vi "AxisUI.vi"(10 "CardNumber":i32, 11 "IO Card Type":T1) -> ()   [LabVIEW 2019]
uses:
  IO Folder/IO_VI/IOCtrl/Ctrl/IO Card_Type.ctl
  Ctrl/right2.ctl
  Ctrl/left2.ctl
  Ctrl/Up2.ctl
  Ctrl/down2.ctl
  Ctrl/Clock2.ctl
  Ctrl/CClock2.ctl
  Ctrl/Teach2.ctl
  Ctrl/Move.ctl
  Ctrl/EmgStop.ctl
  Ctrl/SearchHome.ctl
  <vilib>/Utility/miscctls.llb/LVPointTypeDef.ctl
  LLB/Message/Ctrl/MsgDataInput.ctl
  LLB/Message/Ctrl/MsgPageSelect.ctl
  LLB/Message/Ctrl/LogType.ctl
  IO Folder/IO_VI/IOCtrl/Ctrl/DMC1000B_1 SelectOutput.ctl
  Axis_Class/AxisCard.lvclass
  Axis_Class/DMC 1000B/DMC_1000B.lvclass
  C:/Users/VIC/Desktop/204J1/204J1/System/Function/Axis/Axis_Class/AxisCard.lvclass
  Axis_Class/SubVI/Axis Motion/Axis_Jump Point.vi
  Axis_Class/SubVI/Axis Motion/Axis_Go Point.vi
  Axis_Class/SubVI/Axis Motion/Axis_Go Related.vi
  Axis_Class/SubVI/Axis Motion/Axis_Go Home.vi
  LLB/Commonly VI.lvlib
  LLB/Message/MsgShowAndLog.lvlib
  LLB/DMC1000B/Dmc1000/Dmc1000.lvlib
panel:
  out "Axis Q":refnum<queue>
  out "Axis Q Name":string
  in  "Tab Control":enum32{"Page 1", "Page 2"}(tab)
  in  "Save Button":bool
  out "Actioning":bool
  in  "Btn_EmgStop":T2
  in  "Tab Control 2":enum32{"Control", "PointEdit", "Parameter"}(tab)
  out "Home Finish":T3 caption="Home"
  in  "SearchHome":T4
  in  "JogDistance":cluster{"X":dbl, "Y":dbl, "Z":dbl, "U":dbl}={"X"=10.0, "Y"=10.0, "Z"=10.0, "U"=10.0} caption="寸動距離/JogDistance" {"U" min=0.01 max=100.0 format="%#.3f"; "Z" min=0.01 max=100.0 format="%#.3f"; "Y" min=0.01 max=100.0 format="%#.3f"; "X" min=0.01 max=100.0 format="%#.3f"}
  in  "Btn_Move":T5
  in  "PointSelect":u16(ring) caption="點位選擇/PointSelect" items=["P0 - HM", "P1 - Mark1"]
  in  "Btn_Teach":T6
  in  "Move Action":enum16{"Jump", "Go"}(ring) caption="移動方式/Mode"
  in  "Current Position":cluster{"X":dbl, "Y":dbl, "Z":dbl, "U":dbl} caption="當前位置/Current Position" {"U" format="%#.3f"; "Z" format="%#.3f"; "Y" format="%#.3f"; "X" format="%#.3f"}
  in  "Jog Distance Select":enum32{"Long", "Middle", "Short"}(radio)=enum."Middle" caption="寸動間距選擇(mm)/Jog Distance Select(mm)"
  in  "Jog":T13 caption="寸動/Jog"
  in  "AxisSpeed Basic":T14(array[cluster])=[{"AxisName"="Axis_0", "Accel"=0.5, "Deaccel"=0.5, "Speed"=40000.0, "Sramp"=0.4}, {"AxisName"="Axis_1", "Accel"=0.5, "Deaccel"=0.5, "Speed"=40000.0, "Sramp"=0.4}, {"AxisName"="Axis_2", "Accel"=0.5, "Deaccel"=0.5, "Speed"=40000.0, "Sramp"=0.4}, {"AxisName"="Axis_3", "Accel"=0.5, "Deaccel"=0.5, "Speed"=40000.0, "Sramp"=0.4}]
  in  "RobotPoint":string[][](table)
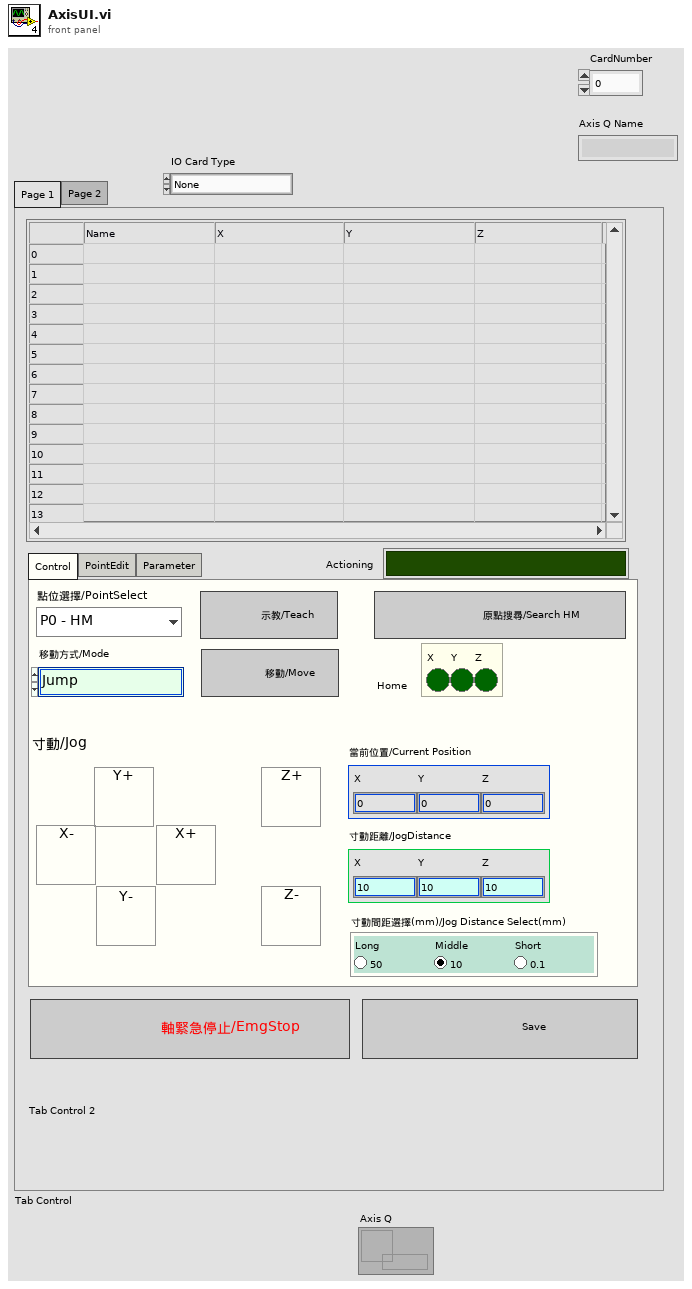
[diagram p1: front panel]
types:
  T1 = typedef "IO Card_Type.ctl" = enum16{"None", "Unidaq32", "6480", "2410C-64", "Zan", "DMC1000B", "16InOut", "Robot", "DMC3600"}
  T2 = typedef "EmgStop.ctl" = bool
  T3 = cluster{"Axis_0":bool, "Axis_1":bool, "Axis_2":bool, "Axis_3":bool}
  T4 = typedef "SearchHome.ctl" = bool
  T5 = typedef "Move.ctl" = bool
  T6 = typedef "Teach2.ctl" = bool
  T7 = typedef "right2.ctl" = bool
  T8 = typedef "left2.ctl" = bool
  T9 = typedef "Up2.ctl" = bool
  T10 = typedef "down2.ctl" = bool
  T11 = typedef "Clock2.ctl" = bool
  T12 = typedef "CClock2.ctl" = bool
  T13 = cluster{"X+":T7, "X-":T8, "Y+":T9, "Y-":T10, "Z+":T9, "Z-":T10, "U+":T11, "U-":T12}
  T14 = cluster{"AxisName":string, "Accel":dbl, "Deaccel":dbl, "Speed":dbl, "Sramp":dbl}[]
  T15 = typedef "LVPointTypeDef.ctl" = cluster{"Horizontal":i16, "Vertical":i16}
  T16 = typedef "MsgDataInput.ctl" = cluster{"MsgPageSelect":T17, "LogType":T18, "Msg":string, "Time":string}
  T17 = typedef "MsgShowAndLog.lvlib/MsgPageSelect.ctl" = enum16{"System", "Comm", "IO", "Action", "Alarm"}
  T18 = typedef "MsgShowAndLog.lvlib/LogType.ctl" = enum16{"Auto", "Manual", "Handshake", "Error"}
  T19 = enum16{"Initial", "Load", "Save", "Read", "WriteSpeed", "WritePoint"}
  T20 = cluster{"Move Action":enum16{"Jump", "Go"}, "RingText.Text":string}
  T21 = cluster{"Move Action":enum16{"Jump", "Go"}, "trimmed string":string}
  T22 = cluster{"[0]":dbl, "[1]":dbl, "[2]":dbl, "[3]":dbl}
  T23 = cluster{"Home Finish[0]":bool, "Home Finish[1]":bool, "Home Finish[2]":bool, "Home Finish[3]":bool}
  T24 = cluster{"Current Position[0]":dbl, "Current Position[1]":dbl, "Current Position[2]":dbl, "Current Position[3]":dbl}
  T25 = typedef "DMC1000B_1 SelectOutput.ctl" = enum16{"M_Out0預備", "M_OUT01蜂鳴器", "M_OUT02紅燈", "M_OUT03綠燈", "M_OUT04黃燈", "M_OUT05上頂固定位氣缸電磁閥", "M_OUT06到料阻擋氣缸電磁閥", "M_OUT07向前機台發出要料#1信號", "M_OUT08向前機台發出要料#2信號", "M_OUT09向後機台發出有料#3信號", "M_OUT10向後機台發出有料#4信號", "M_OUT11接駁台馬達啟動開/關", "M_OUT12接駁台馬達慢速", "M_OUT13抽風機開/關", "M_OUT14上視覺上光源", "M_OUT15DC吹風扇開/關", "M_OUT16Z軸煞車釋放", "M_OUT17", "M_OUT18", "M_OUT19", "M_OUT20", "M_OUT21", "M_OUT22", "M_OUT23", "M_OUT24", "M_OUT25第一軸SEVON1伺服使能信號", "M_OUT26第二軸SEVON2伺服使能信號", "M_OUT27第三軸SEVON3伺服使能信號"}
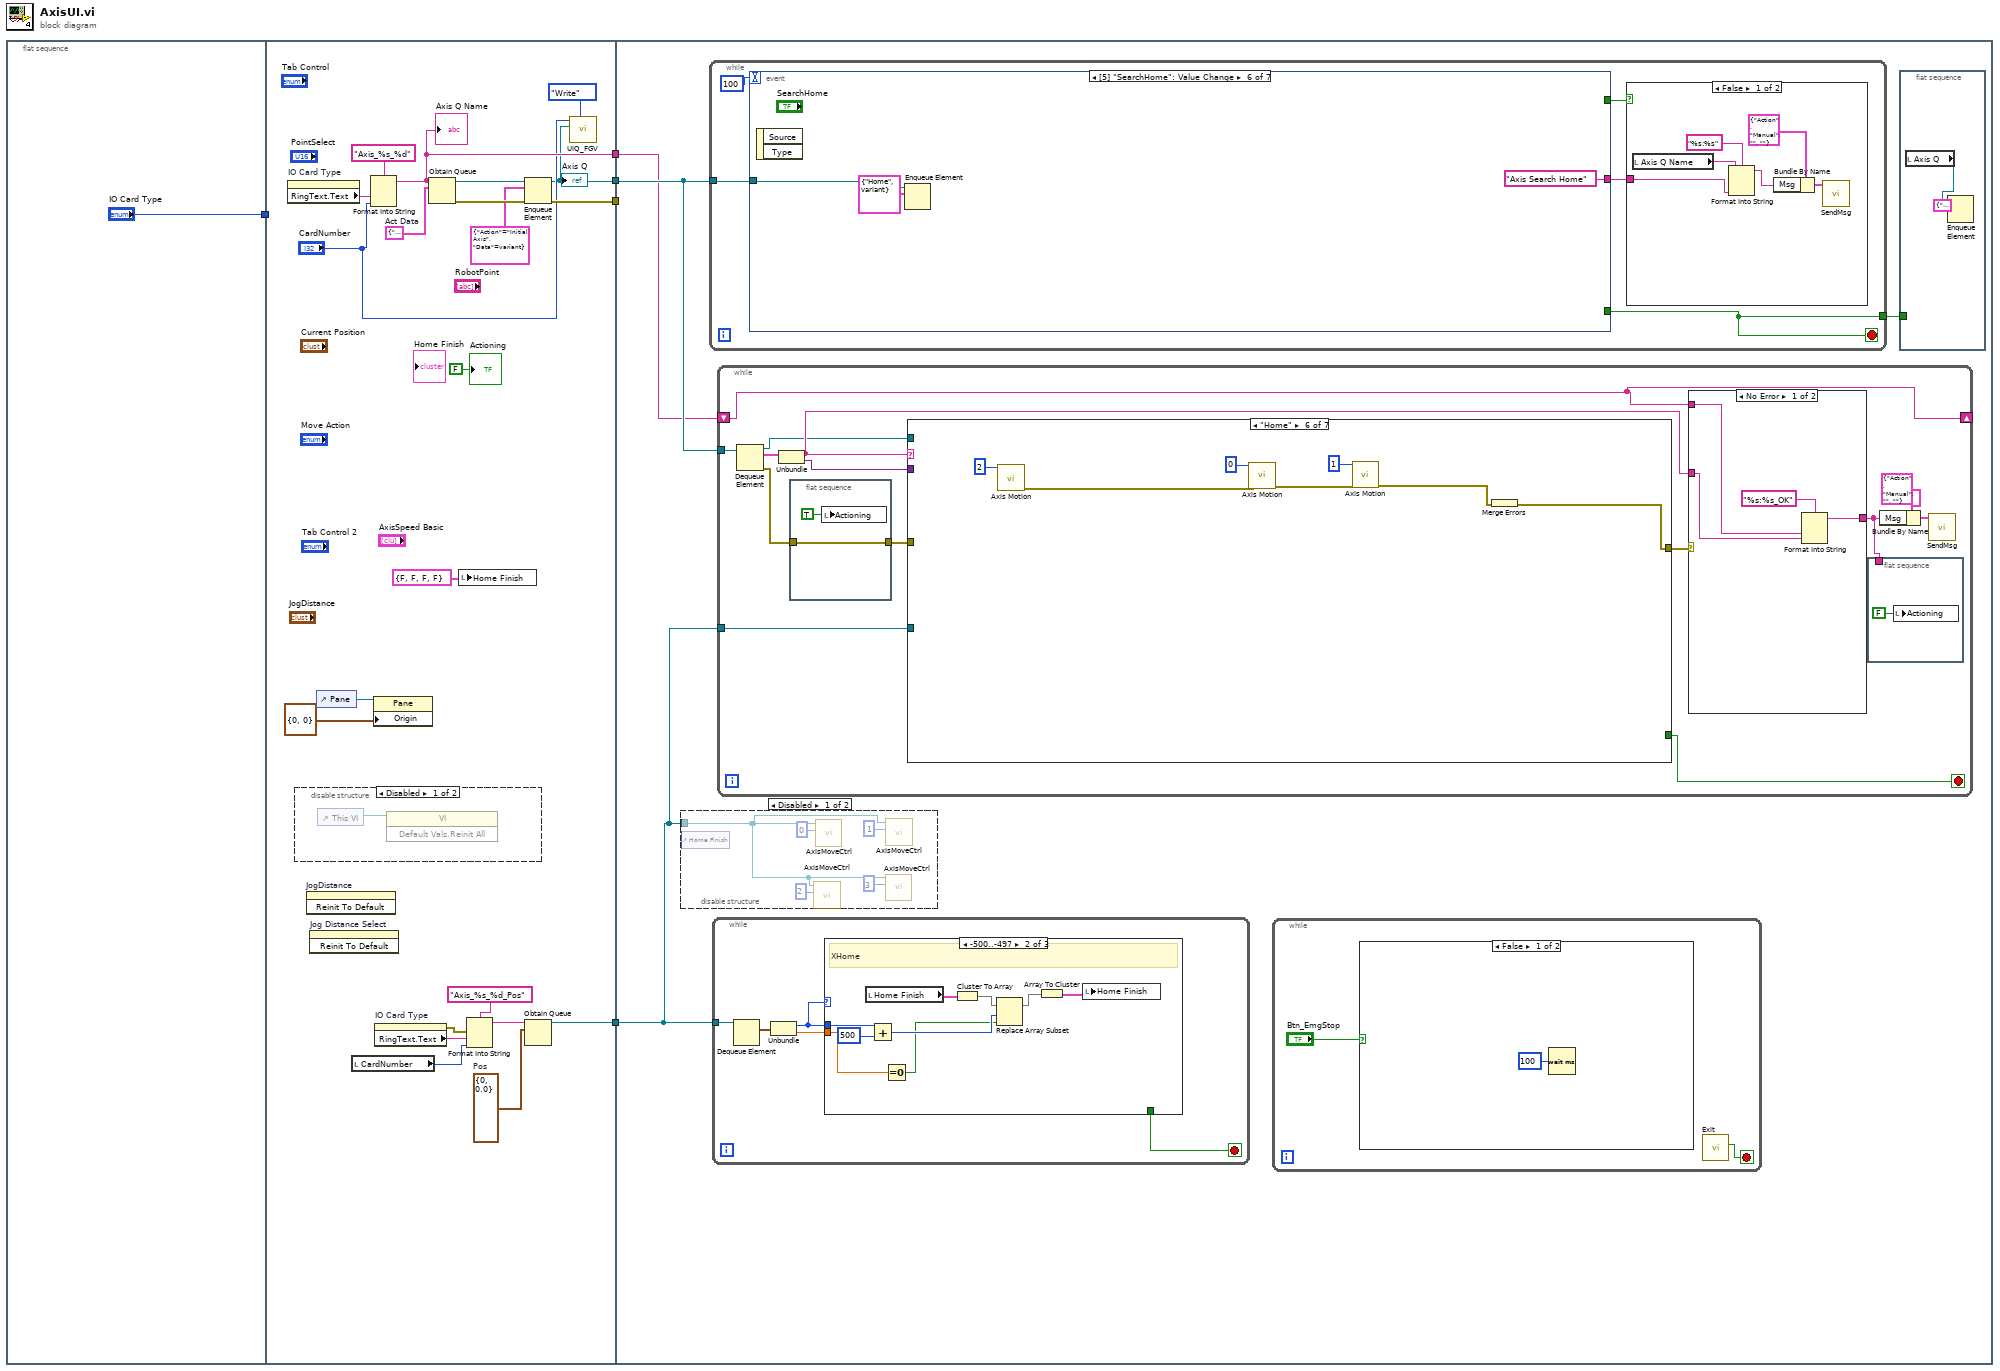
[diagram p0: block diagram]
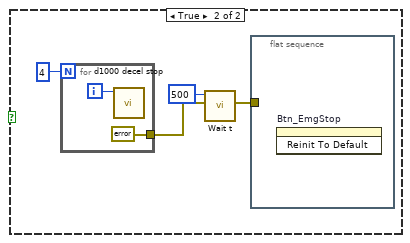
[diagram p4: hidden frame]
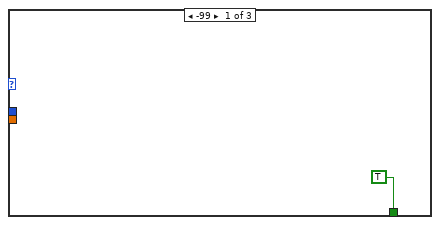
[diagram p5: hidden frame]
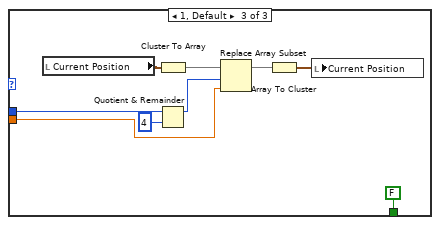
[diagram p6: hidden frame]
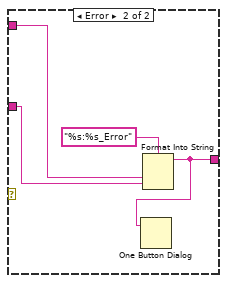
[diagram p7: hidden frame]
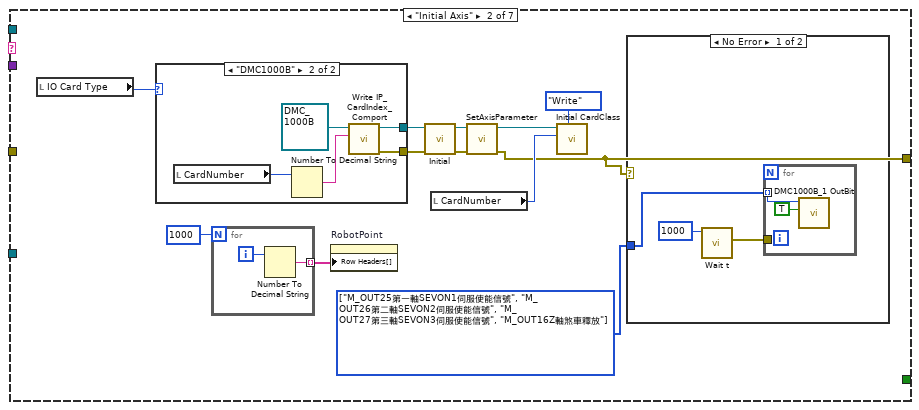
[diagram p9: hidden frame]
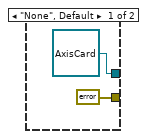
[diagram p11: hidden frame]
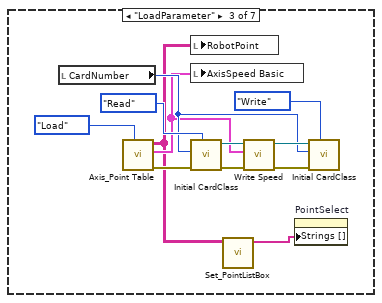
[diagram p12: hidden frame]
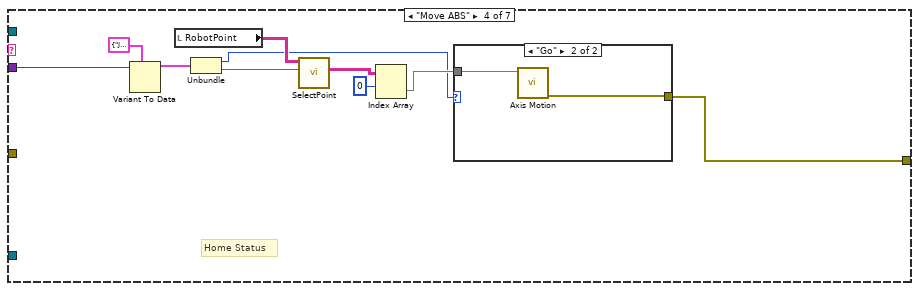
[diagram p13: hidden frame]
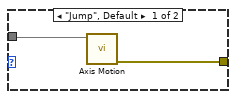
[diagram p14: hidden frame]
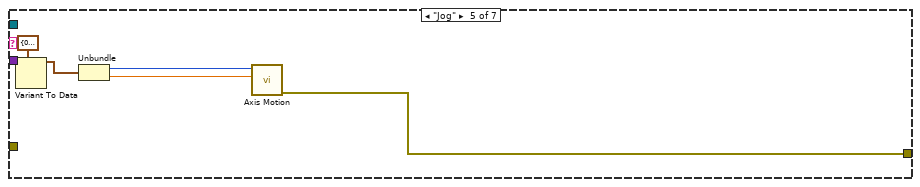
[diagram p15: hidden frame]
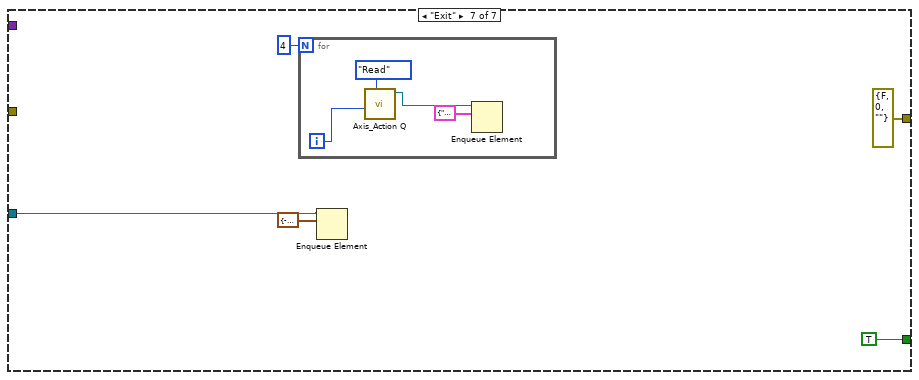
[diagram p16: hidden frame]
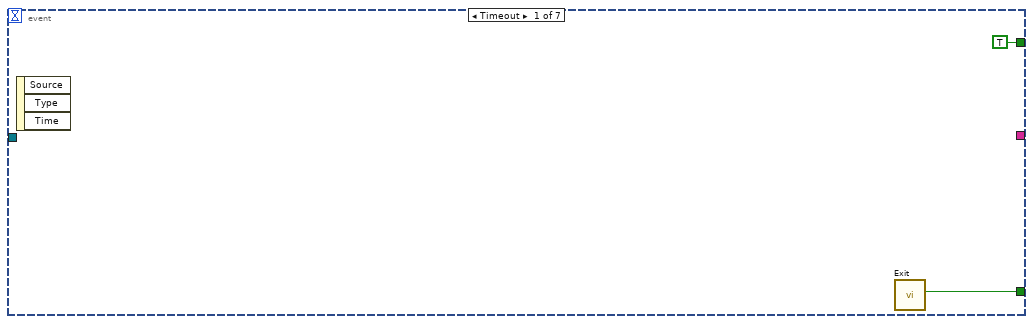
[diagram p18: hidden frame]
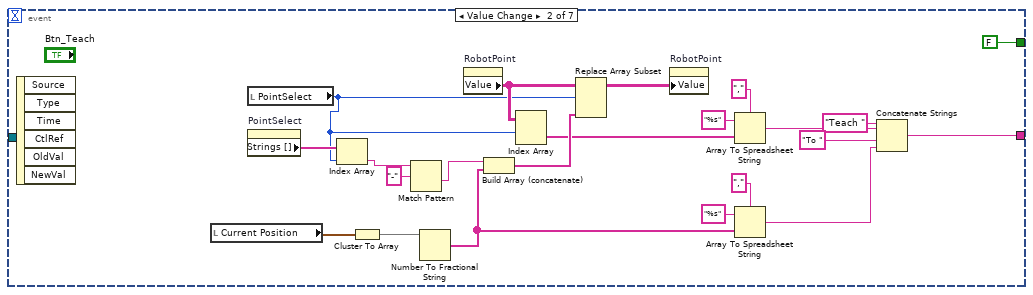
[diagram p19: hidden frame]
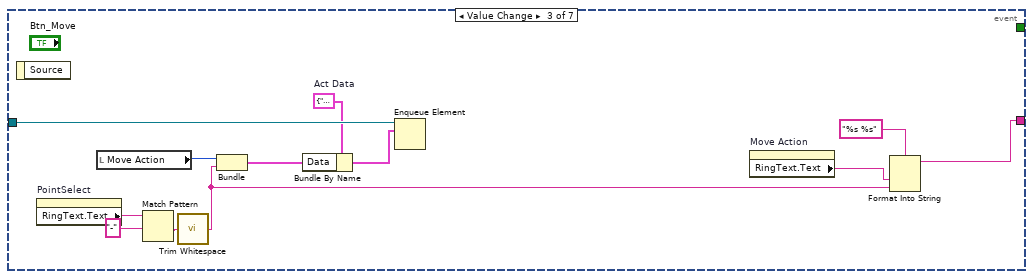
[diagram p20: hidden frame]
diagram:
  n1 = flat-sequence {
    tunnel: ["IO Card Type"] -> w1
    tunnel: [w8] -> w5
    tunnel: [w24] -> w4
    tunnel: [w17] -> w3
    tunnel: [w15] -> w2
    tunnel: w1 -> [_]
    tunnel: w5 -> [w32]
    tunnel: w4 -> [_]
    tunnel: w3 -> [w30]
    tunnel: w2 -> [w31]
    frame #0 {
    }
    frame #1 {
      w16 = cluster{"Action":string, "Data":variant} {"Action"="", "Data"=variant}  # Act Data
      w18 = cluster{"Axis":i32, "Pos":dbl} {"Axis"=0, "Pos"=0.0}  # Pos
      n2 = property on="IO Card Type" class="Enum (strict)"() -> ("RingText.Text"=w26:string)  [unwired: 2 in, 2 out]
      n3 = disable-structure shown="Disabled" {
        frame Disabled {
          n4 = control-ref of="This VI"() -> (w28:refnum<vi>)
          n5 = invoke class="VI" method="Default Vals.Reinit All"(reference=w28) -> ()  [unwired: 2 in, 3 out]
        }
        frame Enabled {
        }
      }
      n6 = invoke on="JogDistance" class="Clust (strict)" method="Reinit To Default"() -> ()  [unwired: 3 in, 3 out]
      n7 = invoke on="Jog Distance Select" class="RadioBtnsControl (strict)" method="Reinit To Default"() -> ()  [unwired: 3 in, 3 out]
      n8 = control-ref of="Pane"() -> (w13:refnum<vi>)
      n9 = local read "CardNumber"() -> (w19:i32)
      n10 = Format Into String(format string="Axis_%s_%d", w26, "CardNumber") -> (resulting string=w15:string)  [unwired: 2 in, 1 out]
      "Axis Q Name" <- w15
      n11 = property class="Pane"(reference=w13, "Origin"=T15 {"Horizontal"=0, "Vertical"=0}) -> ()  [unwired: 1 in, 2 out]
      n12 = property on="IO Card Type" class="Enum (strict)"() -> (error out=w21:errorcluster, "RingText.Text"=w20:string)  [unwired: 2 in, 1 out]
      n13 = Obtain Queue(name (unnamed)=w15, element data type=w16) -> (queue out=w25:refnum<queue>, error out=w24:errorcluster)  [unwired: 3 in, 1 out]
      n14 = local write "Home Finish"(T3 {"Axis_0"=FALSE, "Axis_1"=FALSE, "Axis_2"=FALSE, "Axis_3"=FALSE} ("Home Finish")) -> ()
      n15 = Format Into String(format string="Axis_%s_%d_Pos", error in=w21, w20, w19) -> (resulting string=w23:string)  [unwired: 1 in, 1 out]
      n16 = Enqueue Element(queue=w25, element=cluster{"Action":string, "Data":variant} {"Action"="Initial Axis", "Data"=variant}) -> (queue out=w8:refnum<queue>)  [unwired: 2 in, 2 out]
      "Axis Q" <- w8
      n17 = Obtain Queue(name (unnamed)=w23, element data type=w18) -> (queue out=w17:refnum<queue>)  [unwired: 3 in, 2 out]
      n18 = call "UIQ_FGV.vi"("Enum"=enum16{"Initial", "Write", "Read"}."Write", "DataIn"=w8, "Index"="CardNumber") -> ()  [unwired: 8 in, 1 out]
      "Actioning" <- FALSE ("Actioning")
    }
    frame #2 {
      n19 = disable-structure shown="Disabled" {
        disable-tunnel: w30 -> [w33 _]
        frame Disabled {
          n20 = control-ref of="Home Finish"() -> ()  [unwired: 1 out]
          n21 = call "AxisMoveCtrl.vi"("Axis"=2, "PosQ"=w33) -> ()  [unwired: 10 in]
          n22 = call "AxisMoveCtrl.vi"("Axis"=0, "PosQ"=w33) -> ()  [unwired: 10 in]
          n23 = call "AxisMoveCtrl.vi"("Axis"=3, "PosQ"=w33) -> ()  [unwired: 10 in]
          n24 = call "AxisMoveCtrl.vi"("Axis"=1, "PosQ"=w33) -> ()  [unwired: 10 in]
        }
        frame Enabled {
        }
      }
      n25 = while {
        tunnel: w32 -> [w173]
        tunnel: [w172] -> w29
        stop <- w172 stop-if-true
        n26 = event shown="[5] \"SearchHome\": Value Change" {
          selector: _ -> [_ _ _ _ _ _ _]
          dyn-events: _ -> [_ _ _ _ _ _ _]
          timeout: 100 -> [_ _ _ _ _ _ _]
          tunnel: [w184 _ _ _ _ _ _] -> w172
          tunnel: [_ w188 w211 w221 _ "Axis Search Home" _] -> w175
          tunnel: [TRUE FALSE _ _ _ _ _] -> w174
          tunnel: w173 -> [_ _ w218 w230 _ w241 _]
          event Timeout {
            n27 = event-data() -> ()  [unwired: 1 in, 3 out]
            n28 = call "Exit.vi"() -> ("ExitOut"=w184:bool)  [unwired: 11 in]
          }
          event Value Change {
            n29 = event-data() -> ()  [unwired: 1 in, 6 out]
            n30 = local read "Current Position"() -> (w205:cluster{"X":dbl, "Y":dbl, "Z":dbl, "U":dbl})
            n31 = local read "PointSelect"() -> (w200:u16)
            n32 = property on="PointSelect" class="Ring (strict)"() -> ("Strings []"=w203:string[])  [unwired: 2 in, 2 out]
            n33 = Index Array(array=w203, index=w200) -> (element=w187:string)
            n34 = Cluster To Array(cluster=w205) -> (array=w204:dbl[])
            n35 = Match Pattern(string=w187, regular expression="-") -> (after substring=w186:string)  [unwired: 1 in, 3 out]
            n36 = Number To Fractional String(number=w204) -> (F-format string=w190:string[])  [unwired: 3 in]
            n37 = property on="RobotPoint" class="Tbl (strict)"() -> ("Value"=w201:string[][])  [unwired: 2 in, 2 out]
            n38 = Build Array (concatenate)(w186, w190) -> (w202:string[])
            n39 = Index Array(array=w201, index (row)=w200) -> (element=w199:string[])  [unwired: 1 in]
            n40 = Replace Array Subset(array=w201, new element=w202, index (row)=w200) -> (w206:string[][])  [unwired: 1 in]
            n41 = property on="RobotPoint" class="Tbl (strict)"("Value"=w206) -> ()  [unwired: 2 in, 2 out]
            n42 = Array To Spreadsheet String(delimiter (Tab)=",", array=w199, 3:"%s" ("format string")) -> (spreadsheet string=w194:string)
            n43 = Array To Spreadsheet String(delimiter (Tab)=",", array=w190, 3:"%s" ("format string")) -> (spreadsheet string=w189:string)
            n44 = Concatenate Strings("Teach " ("string"), w194, "To " ("string"), w189) -> (w188:string)
          }
          event Value Change {
            w217 = cluster{"Action":string, "Data":variant} {"Action"="Move ABS", "Data"=variant}  # Act Data
            n45 = event-data() -> ()  [unwired: 1 in, 1 out]
            n46 = property on="PointSelect" class="Ring (strict)"() -> ("RingText.Text"=w213:string)  [unwired: 2 in, 2 out]
            n47 = local read "Move Action"() -> (w215:enum16{"Jump", "Go"})
            n48 = Match Pattern(string=w213, regular expression="-") -> (after substring=w209:string)  [unwired: 1 in, 3 out]
            n49 = call <vilib>:"Trim Whitespace.vi"("string"=w209) -> ("trimmed string"=w207:string)  [unwired: 1 in]
            n50 = Bundle("Move Action"=w215, "trimmed string"=w207) -> (w214:T21)  [unwired: 1 in]
            n51 = Bundle By Name(cluster=w217, "Data"=w214) -> (w216:cluster{"Action":string, "Data":variant})
            n52 = Enqueue Element(queue=w218, element=w216) -> ()  [unwired: 2 in, 3 out]
            n53 = property on="Move Action" class="Enum (strict)"() -> ("RingText.Text"=w208:string)  [unwired: 2 in, 2 out]
            n54 = Format Into String(format string="%s %s", w208, w207) -> (resulting string=w211:string)  [unwired: 2 in, 1 out]
          }
          event "Jog": Value Change {
            n55 = event-data() -> ("NewVal"=w229:T13)  [unwired: 1 in, 1 out]
            n56 = local read "JogDistance"() -> (w227:cluster{"X":dbl, "Y":dbl, "Z":dbl, "U":dbl})
            n57 = Cluster To Array(cluster=w229) -> (array=w228:T12[])
            n58 = Cluster To Array(cluster=w227) -> (array=w226:dbl[])
            n59 = call "Jog btn to Distance.vi"("Distance"=w226, "Jog Btn"=w228) -> ("Distance"=w219:dbl, "Axis"=w220:i32)  [unwired: 7 in, 1 out]
            n60 = Bundle("Axis"=w220, "Distance"=w219) -> (w223:cluster{"Axis":i32, "Distance":dbl})  [unwired: 1 in]
            n61 = Bundle By Name(cluster=cluster{"Action":string, "Data":variant} {"Action"="Jog", "Data"=variant} ("element"), "Data"=w223) -> (w224:cluster{"Action":string, "Data":variant})
            n62 = Enqueue Element(queue=w230, element=w224) -> ()  [unwired: 2 in, 3 out]
            n63 = Format Into String(format string="Axis %d Jog %.3f", w220, w219) -> (resulting string=w221:string)  [unwired: 2 in, 1 out]
          }
          event "Jog Distance Select": Value Change {
            n64 = event-data() -> ()  [unwired: 1 in, 6 out]
            n65 = case shown="\"Short\"" "Jog Distance Select" {
              tunnel: [50.0 10.0 0.1] -> w234
              frame "Long", Default {
              }
              frame "Middle" {
              }
              frame "Short" {
              }
            }
            n66 = Initialize Array(w234, 4 ("dimension size")) -> (w232:dbl[])
            n67 = Array To Cluster(array=w232) -> (cluster=w231:T22)
            n68 = local write "JogDistance"(w231) -> ()
          }
          event Value Change {
            n69 = event-data() -> ()  [unwired: 1 in, 2 out]
            n70 = Enqueue Element(queue=w241, element=cluster{"Action":string, "Data":variant} {"Action"="Home", "Data"=variant}) -> ()  [unwired: 2 in, 3 out]
          }
          event "Save Button": Value Change {
            n71 = event-data() -> ()  [unwired: 1 in, 2 out]
            n72 = local read "RobotPoint"() -> (w244:string[][])
            n73 = local read "AxisSpeed Basic"() -> (w243:T14)
            n74 = call "Axis_Point Table.vi"("Enum"=T19."WritePoint", "PointIn"=w244) -> ("error Out"=w246:errorcluster)  [unwired: 7 in, 2 out]
            n75 = for {
              N: 4 -> [_]
              tunnel: w243 -> [w250] mode=indexing
              shift-right: [w251] -> w245
              shift-left: w246 -> [w252]
              i -> [w249]
              n76 = call "Axis_Point Table.vi"("Enum"=T19."WriteSpeed", "error In"=w252, "AxisData"=w250, "AxisIndex"=w249) -> ("error Out"=w251:errorcluster)  [unwired: 5 in, 2 out]
            }
            n77 = call "Axis_Point Table.vi"("Enum"=T19."Save", "error In"=w245) -> ()  [unwired: 7 in, 3 out]
          }
        }
        n78 = case shown="False" w174 {
          tunnel: w175 -> [w178 _]
          frame False {
            n79 = local read "Axis Q Name"() -> (w180:string)
            n80 = Format Into String(format string="%s:%s", w180, w178) -> (resulting string=w177:string)  [unwired: 2 in, 1 out]
            n81 = Bundle By Name(cluster=T16 {"MsgPageSelect"=enum."Action", "LogType"=enum."Manual", "Msg"="", "Time"=""} ("DataIn"), "Msg"=w177) -> (w182:T16)
            n82 = call "SendMsg.vi"("DataIn"=w182) -> ()  [unwired: 10 in, 1 out]
          }
          frame True {
          }
        }
      }
      n83 = while {
        tunnel: w30 -> [w53]
        stop <- w49 stop-if-true
        n84 = Dequeue Element(queue=w53) -> (element=w52:cluster{"Axis":i32, "Pos":dbl})  [unwired: 2 in, 3 out]
        n85 = Unbundle(w52) -> ("Axis"=w50:i32, "Pos"=w51:dbl)
        n86 = case shown="-500..-497" w50 {
          tunnel: w50 -> [_ w61 w70]
          tunnel: w51 -> [_ w58 w67]
          tunnel: [TRUE _ FALSE] -> w49
          frame -99 {
          }
          frame -500..-497 {
            # "XHome"
            n87 = local read "Home Finish"() -> (w63:T3)
            n88 = Add(x=w61, y=500) -> (x+y=w59:i32)
            n89 = Equal To 0?(x=w58) -> (x = 0?=w57:bool)
            n90 = Cluster To Array(cluster=w63) -> (array=w62:bool[])
            n91 = Replace Array Subset(array=w62, new element=w57, index=w59) -> (w56:bool[])
            n92 = Array To Cluster(array=w56) -> (cluster=w55:T23)
            n93 = local write "Home Finish"(w55) -> ()
          }
          frame 1, Default {
            n94 = local read "Current Position"() -> (w72:cluster{"X":dbl, "Y":dbl, "Z":dbl, "U":dbl})
            n95 = Cluster To Array(cluster=w72) -> (array=w71:dbl[])
            n96 = Quotient & Remainder(x=w70, y=4) -> (x-y*floor(x/y)=w68:i32)  [unwired: 1 out]
            n97 = Replace Array Subset(array=w71, new element=w67, index=w68) -> (w66:dbl[])
            n98 = Array To Cluster(array=w66) -> (cluster=w65:T24)
            n99 = local write "Current Position"(w65) -> ()
          }
        }
      }
      n100 = while {
        tunnel: w32 -> [w86]
        shift-right: [w79] -> _
        shift-left: w31 -> [w79]
        tunnel: w30 -> [w77]
        stop <- w78 stop-if-true
        n101 = Dequeue Element(queue=w86) -> (queue out=w76:refnum<queue>, element=w84:cluster{"Action":string, "Data":variant}, error out=w74:errorcluster)  [unwired: 2 in, 1 out]
        n102 = Unbundle(w84) -> ("Action"=w80:string, "Data"=w83:variant)
        n103 = flat-sequence {
          tunnel: [w89] -> w75
          tunnel: w74 -> [w89]
          frame #0 {
            n104 = local write "Actioning"(TRUE ("Actioning")) -> ()
          }
        }
        n105 = case shown="\"Home\"" w80 {
          tunnel: [_ w99 _ w136 w150 w159 errorcluster {"status"=FALSE, "code"=0, "source"=""} ("error IO")] -> w85
          tunnel: w83 -> [_ _ _ w144 w154 _ _]
          tunnel: [_ _ _ _ _ _ TRUE] -> w78
          tunnel: w77 -> [_ _ _ _ _ _ w164]
          tunnel: w76 -> [_ _ _ _ _ _ _]
          tunnel: w75 -> [_ _ _ _ _ _ _]
          frame "False", Default {
          }
          frame "Initial Axis" {
            w98 = T25[] [enum."M_OUT25第一軸SEVON1伺服使能信號", enum."M_OUT26第二軸SEVON2伺服使能信號", enum."M_OUT27第三軸SEVON3伺服使能信號", enum."M_OUT16Z軸煞車釋放"] items=["M_Out0預備", "M_OUT01蜂鳴器", "M_OUT02紅燈", "M_OUT03綠燈", "M_OUT04黃燈", "M_OUT05上頂固定位氣缸電磁閥", "M_OUT06到料阻擋氣缸電磁閥", "M_OUT07向前機台發出要料#1信號", "M_OUT08向前機台發出要料#2信號", "M_OUT09向後機台發出有料#3信號", "M_OUT10向後機台發出有料#4信號", "M_OUT11接駁台馬達啟動開/關", "M_OUT12接駁台馬達慢速", "M_OUT13抽風機開/關", "M_OUT14上視覺上光源", "M_OUT15DC吹風扇開/關", "M_OUT16Z軸煞車釋放", "M_OUT17", "M_OUT18", "M_OUT19", "M_OUT20", "M_OUT21", "M_OUT22", "M_OUT23", "M_OUT24", "M_OUT25第一軸SEVON1伺服使能信號", "M_OUT26第二軸SEVON2伺服使能信號", "M_OUT27第三軸SEVON3伺服使能信號"]
            n106 = local read "IO Card Type"() -> (w109:T1)
            n107 = case shown="\"DMC1000B\"" w109 {
              tunnel: [refnum<class "AxisCard.lvclass"> refnum ("AxisCard.lvclass") w120] -> w108
              tunnel: [errorcluster {"status"=FALSE, "code"=0, "source"=""} ("error out") w119] -> w107
              frame "None", Default {
              }
              frame "DMC1000B" {
                n108 = local read "CardNumber"() -> (w122:i32)
                n109 = Number To Decimal String(number=w122) -> (decimal integer string=w121:string)  [unwired: 1 in]
                n110 = call-dynamic "Write IP_CardIndex_Comport.vi"("IP/CardIndex/Comport"=w121, "AxisCard in"=refnum<class "DMC_1000B.lvclass"> refnum ("DMC_1000B.lvclass")) -> ("error out"=w119:errorcluster, "AxisCard out"=w120:refnum<class "DMC_1000B.lvclass">)  [unwired: 8 in]
              }
            }
            n111 = for {
              N: 1000 -> [_]
              tunnel: [w115] -> w100 mode=indexing
              i -> [w116]
              n112 = Number To Decimal String(number=w116) -> (decimal integer string=w115:string)  [unwired: 1 in]
            }
            n113 = property on="RobotPoint" class="Tbl (strict)"("Row Headers[]"=w100) -> ()  [unwired: 2 in, 2 out]
            n114 = call-dynamic "Initial.vi"("error in (no error)"=w107, "AxisCard in"=w108) -> ("error out"=w105:errorcluster, "AxisCard out"=w106:refnum<class "AxisCard.lvclass">)  [unwired: 8 in]
            n115 = local read "CardNumber"() -> (w102:i32)
            n116 = call-dynamic "SetAxisParameter.vi"("error in (no error)"=w105, "AxisCard in"=w106) -> ("error out"=w99:errorcluster, "AxisCard out"=w104:refnum<class "AxisCard.lvclass">)  [unwired: 8 in]
            n117 = call "Initial CardClass.vi"("Enum"=enum16{"Initial", "Write", "Read", "Exit"}."Write", "Card Number"=w102, "ClassIn"=w104) -> ()  [unwired: 7 in, 2 out]
            n118 = case shown="No Error" w99 {
              tunnel: w98 -> [w112 _]
              frame No Error {
                n119 = call "Wait t.vi"("wait(ms)"=u32 1000) -> ("error out"=w111:errorcluster)  [unwired: 10 in]
                n120 = for {
                  tunnel: w112 -> [w113] mode=indexing
                  tunnel: w111 -> [_]
                  n121 = call "DMC1000B_1 OutBit.vi"("BL"=TRUE, "IO_Output_1 Select"=w113) -> ()  [unwired: 9 in, 1 out]
                }
              }
              frame Error {
              }
            }
          }
          frame "LoadParameter" {
            n122 = local read "CardNumber"() -> (w131:i32)
            n123 = call "Axis_Point Table.vi"("Enum"=T19."Load") -> ("error Out"=w126:errorcluster, "AxisSpeed Basic"=w129:T14, "RobotPoint"=w125:string[][])  [unwired: 8 in]
            n124 = local write "RobotPoint"(w125) -> ()
            n125 = local write "AxisSpeed Basic"(w129) -> ()
            n126 = call "Initial CardClass.vi"("Enum"=enum16{"Initial", "Write", "Read", "Exit"}."Read", "error in"=w126, "Card Number"=w131) -> ("error Out"=w128:errorcluster, "DataOut"=w134:refnum<class "AxisCard.lvclass">)  [unwired: 7 in]
            n127 = call "Set_PointListBox.vi"("Table"=w125) -> ("Point"=w124:string[])  [unwired: 10 in]
            n128 = call-dynamic "Write Speed.vi"("error in (no error)"=w128, "AxisSpeed"=w129, "AxisCard in"=w134) -> ("error out"=w127:errorcluster, "AxisCard out"=w133:refnum<class "AxisCard.lvclass">)  [unwired: 7 in]
            n129 = property on="PointSelect" class="Ring (strict)"("Strings []"=w124) -> ()  [unwired: 2 in, 2 out]
            n130 = call "Initial CardClass.vi"("Enum"=enum16{"Initial", "Write", "Read", "Exit"}."Write", "error in"=w127, "Card Number"=w131, "ClassIn"=w133) -> ()  [unwired: 6 in, 2 out]
          }
          frame "Move ABS" {
            # "Home Status"
            n131 = Variant To Data(type=T20 {"Move Action"=enum."Jump", "RingText.Text"=""} ("output cluster"), Variant=w144) -> (data=w143:T20)  [unwired: 1 in, 1 out]
            n132 = local read "RobotPoint"() -> (w142:string[][])
            n133 = Unbundle(w143) -> ("Move Action"=w137:enum16{"Jump", "Go"}, "RingText.Text"=w141:string)
            n134 = call "SelectPoint.vi"("PointName"=w141, "RobotPointsTableIn"=w142) -> ("RobotPointsOut"=w140:string[][])  [unwired: 7 in, 2 out]
            n135 = Index Array(array=w140, index (row)=0) -> (element=w138:string[])  [unwired: 1 in]
            n136 = case shown="\"Go\"" w137 {
              tunnel: w138 -> [w146 w149]
              tunnel: [w147 w148] -> w136
              frame "Jump", Default {
                n137 = call-poly "Axis Motion.vi"("RobotPoints in"=w146) -> ("error out"=w147:errorcluster)  [unwired: 10 in]
              }
              frame "Go" {
                n138 = call-poly "Axis Motion.vi"("RobotPoints in"=w149) -> ("error out"=w148:errorcluster)  [unwired: 10 in]
              }
            }
          }
          frame "Jog" {
            n139 = Variant To Data(type=cluster{"Axis":i32, "Distance":dbl} {"Axis"=0, "Distance"=0.0} ("output cluster"), Variant=w154) -> (data=w153:cluster{"Axis":i32, "Distance":dbl})  [unwired: 1 in, 1 out]
            n140 = Unbundle(w153) -> ("Axis"=w152:i32, "Distance"=w151:dbl)
            n141 = call-poly "Axis Motion.vi"("Distance"=w151, "Axis Index"=w152) -> ("error"=w150:errorcluster)  [unwired: 9 in]
          }
          frame "Home" {
            n142 = call-poly "Axis Motion.vi"("Axis Index"=2) -> ("error"=w156:errorcluster)  [unwired: 10 in]
            n143 = call-poly "Axis Motion.vi"("error in"=w156, "Axis Index"=0) -> ("error"=w158:errorcluster)  [unwired: 9 in]
            n144 = call-poly "Axis Motion.vi"("error in"=w158, "Axis Index"=1) -> ("error"=w157:errorcluster)  [unwired: 9 in]
            n145 = Merge Errors(w157) -> (w159:errorcluster)
          }
          frame "Exit" {
            n146 = for {
              N: 4 -> [_]
              i -> [w170]
              n147 = call "Axis_Action Q.vi"("Enum"=enum16{"Initial", "Write", "Read"}."Read", "Axis Index"=w170) -> ("Axis ActQ Out"=w169:refnum<queue>)  [unwired: 7 in, 2 out]
              n148 = Enqueue Element(queue=w169, element=cluster{"Action":string, "Data":variant} {"Action"="Exit", "Data"=variant}) -> ()  [unwired: 2 in, 3 out]
            }
            n149 = Enqueue Element(queue=w164, element=cluster{"Axis":i32, "Pos":dbl} {"Axis"=-99, "Pos"=0.0}) -> ()  [unwired: 2 in, 3 out]
          }
        }
        n150 = case shown="No Error" w85 {
          tunnel: w80 -> [w92 w96]
          tunnel: [w91 w94] -> w73
          tunnel: w79 -> [w90 w95]
          frame No Error {
            n151 = Format Into String(format string="%s:%s_OK", w90, w92) -> (resulting string=w91:string)  [unwired: 2 in, 1 out]
          }
          frame Error {
            n152 = Format Into String(format string="%s:%s_Error", w95, w96) -> (resulting string=w94:string)  [unwired: 2 in, 1 out]
            n153 = One Button Dialog(message=w94) -> ()  [unwired: 1 in, 1 out]
          }
        }
        n154 = flat-sequence {
          tunnel: w73 -> [_]
          frame #0 {
            n155 = local write "Actioning"(FALSE ("Actioning")) -> ()
          }
        }
        n156 = Bundle By Name(cluster=T16 {"MsgPageSelect"=enum."Action", "LogType"=enum."Manual", "Msg"="", "Time"=""} ("DataIn"), "Msg"=w73) -> (w82:T16)
        n157 = call "SendMsg.vi"("DataIn"=w82) -> ()  [unwired: 10 in, 1 out]
      }
      n158 = while {
        stop <- w40 stop-if-true
        n159 = case shown="False" "Btn_EmgStop" {
          frame False {
            n160 = Wait (ms)(milliseconds to wait=u32 100) -> ()  [unwired: 1 out]
          }
          frame True {
            n161 = for {
              N: 4 -> [_]
              tunnel: [errorcluster {"status"=FALSE, "code"=0, "source"=""} ("error constant")] -> w44
              i -> [w48]
              n162 = call "d1000 decel stop.vi"("axis"=w48) -> ()  [unwired: 10 in, 1 out]
            }
            n163 = call "Wait t.vi"("error in"=w44, "wait(ms)"=u32 500) -> ("error out"=w43:errorcluster)  [unwired: 9 in]
            n164 = flat-sequence {
              tunnel: w43 -> [_]
              frame #0 {
                n165 = invoke on="Btn_EmgStop" class="Bool" method="Reinit To Default"() -> ()  [unwired: 3 in, 3 out]
              }
            }
          }
        }
        n166 = call "Exit.vi"() -> ("ExitOut"=w40:bool)  [unwired: 11 in]
      }
      n167 = flat-sequence {
        tunnel: w29 -> [_]
        frame #0 {
          n168 = local read "Axis Q"() -> (w39:refnum<queue>)
          n169 = Enqueue Element(queue=w39, element=cluster{"Action":string, "Data":variant} {"Action"="Exit", "Data"=variant}) -> ()  [unwired: 2 in, 3 out]
        }
      }
    }
  }
